vi "Change Message Visibility.vi"(8 "error in (no error)":errorcluster, 9 "Visibility Timeout":i32, 10 "Receipt Handle":string, 11 "SQS in":refnum<class "Queue.lvclass">) -> (0 "error out":errorcluster, 3 "SQS out":refnum<class "Queue.lvclass">)   [LabVIEW 2015, in "NI_AWS_SQS.lvlib" / "Queue.lvclass"]
doc: "Changes the visibility timeout of a specified message in a queue to a new value. The maximum allowed timeout value is 12 hours. Thus, you can't extend the timeout of a message in an existing queue to more than a total visibility timeout of 12 hours. For more information, see Visibility Timeout in the Amazon SQS Developer Guide.\n\nFor example, you have a message and with the default visibility timeout of 5 minutes. After 3 minutes, you call ChangeMessageVisiblity with a timeout of 10 minutes. At that time, the timeout for the message is extended by 10 minutes beyond the time of the ChangeMessageVisibility action. This results in a total visibility timeout of 13 minutes. You can continue to call the ChangeMessageVisibility to extend the visibility timeout to a maximum of 12 hours. If you try to extend the visibility timeout beyond 12 hours, your request is rejected.\n\nA message is considered to be in flight after it's received from a queue by a consumer, but not yet deleted from the queue.\n\nFor standard queues, there can be a maximum of 120,000 inflight messages per queue. If you reach this limit, Amazon SQS returns the OverLimit error message. To avoid reaching the limit, you should delete messages from the queue after they're processed. You can also increase the number of queues you use to process your messages.\n\nFor FIFO queues, there can be a maximum of 20,000 inflight messages per queue. If you reach this limit, Amazon SQS returns no error messages.\n\nImportant\nIf you attempt to set the VisibilityTimeout to a value greater than the maximum time left, Amazon SQS returns an error. Amazon SQS doesn't automatically recalculate and increase the timeout to the maximum remaining time.\nUnlike with a queue, when you change the visibility timeout for a specific message the timeout value is applied immediately but isn't saved in memory for that message. If you don't delete a message after it is received, the visibility timeout for the message reverts to the original timeout value (not to the value you set using the ChangeMessageVisibility action) the next time the message is received."
uses:
  Queue.lvclass
  Core/HTTP Request/Name Value Pair.ctl
  Core/HTTP Request/Request Options.ctl
  Core/HTTP Request/Region handling.ctl
  Core/HTTP Request/URL formatting.ctl
  Queue.lvclass/Queue.ctl
  Read Account Number.vi
  Read Name.vi
  Core/HTTP Request/HTTP Request.lvclass
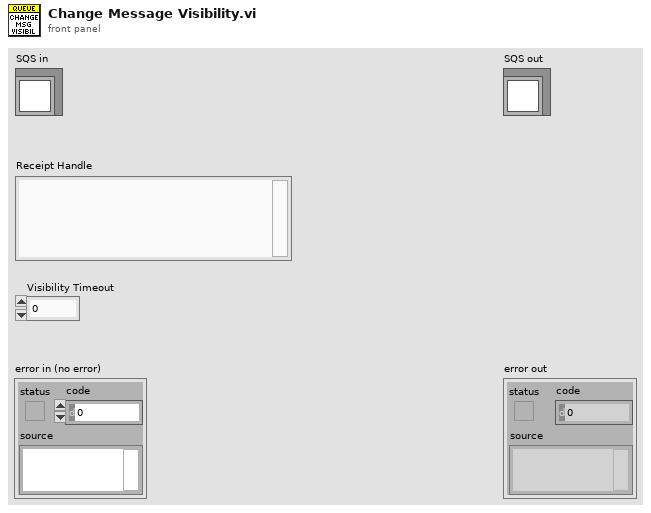
[diagram p1: front panel]
types:
  T1 = typedef "NI_AWS_Core.lvlib/HTTP Request.lvclass/Name Value Pair.ctl" = cluster{"name":string, "value":string}
  T2 = typedef "NI_AWS_Core.lvlib/HTTP Request.lvclass/Request Options.ctl" = cluster{"request headers":T1[], "request parameters":T1[], "request body":string, "region handling":T3, "URL formatting":T4}
  T3 = typedef "NI_AWS_Core.lvlib/HTTP Request.lvclass/Region handling.ctl" = enum16{"use region everywhere", "use region (authentication only)", "use region (URL only)", "ignore region everwhere"}
  T4 = typedef "NI_AWS_Core.lvlib/HTTP Request.lvclass/URL formatting.ctl" = enum16{"region-", "region."}
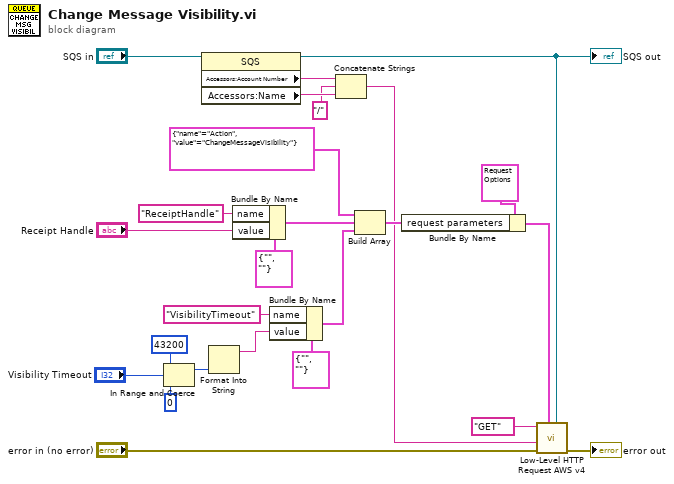
[diagram p0: block diagram]
diagram:
  n1 = In Range and Coerce(upper limit=43200, x="Visibility Timeout", lower limit=0) -> (coerced(x)=w2:i32)  [unwired: 1 out]
  n2 = property class="SQS"(reference="SQS in") -> (reference out=w18:refnum<class "Queue.lvclass">, "Accessors:Account Number"=w17:string, "Accessors:Name"=w16:string)  [unwired: 1 in, 1 out]
  "SQS out" <- w18
  n3 = Format Into String(w2) -> (resulting string=w1:string)  [unwired: 3 in, 1 out]
  n4 = Bundle By Name(cluster=T1 {"name"="", "value"=""} ("element"), "name"="ReceiptHandle", "value"="Receipt Handle") -> (w11:T1)
  n5 = Bundle By Name(cluster=T1 {"name"="", "value"=""} ("element"), "name"="VisibilityTimeout", "value"=w1) -> (w6:T1)
  n6 = Concatenate Strings(w17, "/", w16) -> (w14:string)
  n7 = Build Array(T1 {"name"="Action", "value"="ChangeMessageVisibility"} ("Cluster"), w11, w6) -> (w19:T1[])
  n8 = Bundle By Name(cluster=T2 {"request headers"=[], "request parameters"=[{"name"="Action", "value"="ListQueues"}], "request body"="", "region handling"=enum."use region everywhere", "URL formatting"=enum."region."} ("Request Options"), "request parameters"=w19) -> (w20:T2)
  n9 = call "Low-Level HTTP Request AWS v4.vi"("AWS Core"=w18, "Request Options"=w20, "error in (no error)"="error in (no error)", "URL Suffix"=w14, "HTTP-Verb"="GET") -> ("error out"=→"error out":errorcluster)  [unwired: 4 in, 2 out]
